vi "VI Auto Kalibrieren.vi"() -> ()   [LabVIEW 2020, in "Auto Kalibrieren.lvlib"]
uses:
  Auto Kalibrieren.lvlib
  Visualisierungs Elemente/Button.ctl
  Visualisierungs Elemente/String - Ausgabefeld.ctl
  Visualisierungs Elemente/Zahlen-Ausgabefeld.ctl
  Funktionstasten/Funktionstasten-Aktion.ctl
  Funktionstasten/Zustaende.ctl
  Aktionen FGV Zustand Kalibrierung.ctl
  Funktionstasten/Freigabe Aktionen.ctl
  Seiten/FT-IR/FGV FT-IR Gasliste Aktionen.ctl
  Aktionen Timeout.ctl
  Analysator Definition/FGV Analysator Definition Aktionen.ctl
  Status Analysatoren/Aktion Status Analysatoren.ctl
  Aktion FGV CalZustand.ctl
  Seiten/CalGas Aufschaltung/FGV CalGas Aktionen.ctl
  Funktionstasten/Aktionen Zustaende Loggen.ctl
  Sprachverwaltung/FGV Aktion Tabelle zerlegen.ctl
  Aktion FGV Autokal GT.ctl
  Aktionen FID kalibrieren.ctl
  Aktionen FT-IR Kalibrieren.ctl
  Seiten/FT-IR/TOOLweb Interface Library/Trigger Aktionen.ctl
  Aktionen PMA kalibrieren.ctl
  Messdaten/Aktionen FGV Messdaten.ctl
  Seiten/EL3000/Allgemeine VI/FGV Uras26 Aktion.ctl
  Aktionen Zeitstempel speichern.ctl
  Stoerungen/FGV Stoerung aufnehmen Aktion.ctl
  Seiten/FT-IR/ReadLabFile/Aktionen Lab File.ctl
  Stoerungen/Stoerungen Messgeraet/Aktionen Kommunikation Stoerung.ctl
  SysLog/SysLog Interface.ctl
  Seiten/FT-IR/TOOLweb Interface Library/TOOLweb Interface.lvlib
  Seiten/FT-IR/TOOLweb Interface Library/Typdefinitionen.lvlib
  Funktionstasten/Funktionstasten.lvlib
  Allgemein/allgemeine Sub-VIs.lvlib
  Seiten/FT-IR/FT-IR.lvlib
  Messdaten/Messdaten.lvlib
  Analysator Definition/Analysator Definition.lvlib
  Seiten/EL3000/PMA/Kalibrieren/Kalibrieren.lvlib
  Seiten/EL3000/Allgemeine VI/Allgemeine VI.lvlib
  Status Analysatoren/Status Analysatoren.lvlib
  Seiten/EL3000/FID/FID Kalibrierung/FID Kalibrierung.lvlib
  Seiten/CalGas Aufschaltung/CalGas Aufschaltung.lvlib
  SysLog/SysLog.lvlib
  Stoerungen/Stoerungen.lvlib
  Seiten/FT-IR/ReadLabFile/Read Lab File.lvlib
  Linearisierung V2/Linearisierung v2.lvlib
  Sprachverwaltung/Sprachverwaltung.lvlib
panel:
  out "Endpunktgas Konzentration O2:":T1 caption="%" format="%.2f"
  out "Endpunktgas Konzentration THC:":T1 caption="ppm" format="%.2f"
  out "Zustand FID THC":T2
  out "Dev THC":sgl caption="ppm" format="%.2f"
  out "Rohwert THC":T1 caption="ppm" format="%.2f"
  out "Dev CH4":sgl caption="ppm" format="%.2f"
  out "Raw value CH4":T1 caption="ppm" format="%.2f"
  out "Zustand FID":T2
  out "Zustand PMA":T2
  out "Dev O2":sgl caption="Konzentration" format="%.2f"
  out "Rohwert O2":T1 caption="%" format="%.2f"
  out "Zustand FT-IR":T2
  out "Dev H2O":sgl caption="Konzentration" format="%.2f"
  out "Dev CO2":sgl caption="Konzentration" format="%.2f"
  out "CO2":T1 caption="%" format="%.2f"
  out "H2O":T1 caption="%" format="%.2f"
  out "Zeit:":T1 caption="Zeit"
  in  "ABBRECHEN":T3
  # "Auto Kalibrierung"
  # "sec"
  # "FID CH4:"
  # "FID THC:"
  # "Dev.:"
  # "Dev.:"
  # "Dev.:"
  # "%"
  # "PMD:"
  # "Dev.:"
  # "%"
  # "Dev.:"
  # "%"
  # "FT-IR:"
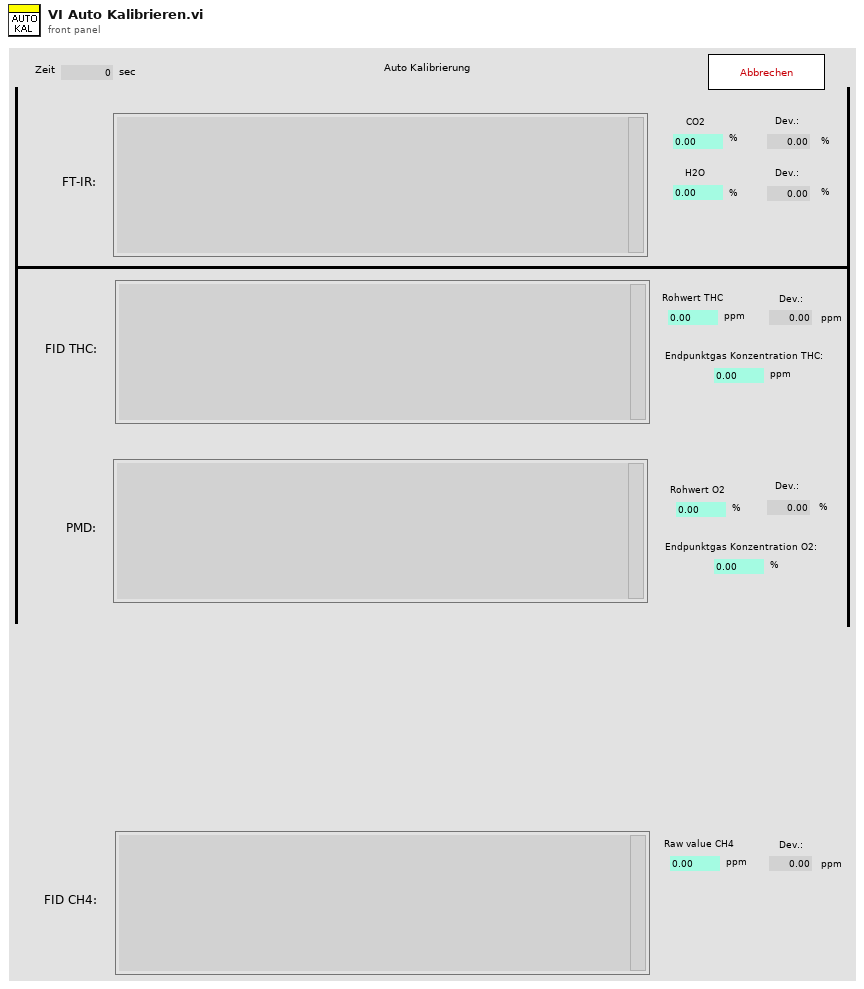
[diagram p1: front panel]
types:
  T1 = typedef "Zahlen-Ausgabefeld.ctl" = sgl
  T2 = typedef "String - Ausgabefeld.ctl" = string
  T3 = typedef "Button.ctl" = bool
  T4 = typedef "Funktionstasten.lvlib/Zustaende.ctl" = enum16{"Standby", "Pause", "Eco", "Messen", "Kalibrieren", "Spülen Filter", "Spülen Leitung", "Umgebungsluft", "0-Gas", "Cal-Gas", "CG zu PNS", "-------------", "Init 1", "Init 2", "Init 3", "Init 4", "Messen vorbereiten", "Messen durchführen", "Exit"}
  T5 = typedef "Funktionstasten.lvlib/Funktionstasten-Aktion.ctl" = enum16{"Initialisieren", "Zustand setzen", "Taste gedrückt", "Fehler speichern", "Lesen", "Manuell", "Remote", "Bitparallel", "Samplepoint", "Zeit Prüfen", "reset Umschalten"}
  T6 = typedef "Sprachverwaltung.lvlib/FGV Aktion Tabelle zerlegen.ctl" = enum16{"laden", "vereinzeln", "speichern"}
  T7 = typedef "Funktionstasten.lvlib/Aktionen Zustaende Loggen.ctl" = enum16{"lesen", "schreiben", "löschen", "init"}
  T8 = typedef "CalGas Aufschaltung.lvlib/FGV CalGas Aktionen.ctl" = enum16{"lesen", "Analysator Auswahl", "Def.CalGas", "Aufschaltung CalGas", "laden", "speichern", "KAL extrahieren"}
  T9 = typedef "Auto Kalibrieren.lvlib/Aktion FGV CalZustand.ctl" = enum16{"lesen", "Cal FTIR", "Cal FID CH4", "Cal PMA", "init", "Cal FID THC", "THC CG Eingang"}
  T10 = typedef "Status Analysatoren.lvlib/Aktion Status Analysatoren.ctl" = enum16{"lesen", "initialisieren", "Analysatoren aktiv", "FTIR Fehler", "FID Fehler", "PMA Fehler", "Felder einfärben"}
  T11 = typedef "Analysator Definition.lvlib/FGV Analysator Definition Aktionen.ctl" = enum16{"lesen", "MB setzen", "MB KAL setzen", "laden"}
  T12 = typedef "Auto Kalibrieren.lvlib/Aktionen Timeout.ctl" = enum16{"lesen", "init", "prüfen"}
  T13 = typedef "FT-IR.lvlib/FGV FT-IR Gasliste Aktionen.ctl" = enum16{"lesen", "Gasliste FT-IR", "Gasliste ausgelesen", "laden", "speichern", "löschen"}
  T14 = typedef "Funktionstasten.lvlib/Freigabe Aktionen.ctl" = enum16{"prüfen", "Freigabe?", "lesen"}
  T15 = typedef "Auto Kalibrieren.lvlib/Aktionen FGV Zustand Kalibrierung.ctl" = enum16{"lesen", "LÖSCHEN", "Hintergrund fertig", "Nullpunkt NDIR CO lo", "Endpunkt NDIR CO lo", "Nullpunkt NDIR CO hi", "Endpunkt NDIR CO hi", "Nullpunkt NDIR CO2 lo", "Endpunkt NDIR CO2 lo", "Nullpunkt FID CH4", "Endpunkt FID CH4", "Nullpunkt FID THC", "Endpunkt FID THC", "Nullpunkt PMA", "Endpunkt PMA", "Fehler FT-IR", "Fehler NDIR lo", "Fehler FID CH4", "Fehler FID THC", "Fehler PMA", "TIMEOUT"}
  T16 = typedef "Auto Kalibrieren.lvlib/Aktion FGV Autokal GT.ctl" = enum16{"lesen", "Autokal GT", "Referenz Start"}
  T17 = typedef "Status Analysatoren.lvlib/Status.ctl" = cluster{"FT-IR aktiv":bool, "FT-IR Fehler":bool, "FID aktiv":bool, "FID Fehler":bool, "PMA aktiv":bool, "PMA Fehler":bool}
  T18 = typedef "Analysator Definition.lvlib/Betriebsdaten Komponente.ctl" = cluster{"Namen":string[], "MB Namen":string[], "Einheit":string, "MB Aktuell":u16, "MB Endwert":u16, "CalGase":u16[], "MB für KAL":u16[], "CG für KAL":u16[]}
  T19 = typedef "ABB-EL3000.lvlib/Allgemeine VI.lvlib/FGV Uras26 Aktion.ctl" = enum16{"lesen", "CAL-Daten laden", "Messen", "Kalibrieren vorbereiten", "Kalibrieren", "CAL-Daten speichern", "Toleranz schreiben", "CAL-Daten kopieren"}
  T20 = typedef "Messdaten.lvlib/Aktionen FGV Messdaten.ctl" = enum16{"lesen", "schreiben", "löschen", "Mittelwerte", "Komponente"}
  T21 = typedef "Auto Kalibrieren.lvlib/Aktionen Zeitstempel speichern.ctl" = enum16{"lesen", "Zeitstempel NEU", "laden", "speichern"}
  T22 = typedef "CalGas Aufschaltung.lvlib/Definition CalGas Anzeige.ctl" = cluster{"Namen":T23, "Werte":T25, "Werte 2":T25, "Einheit":T27, "Messbereiche":T29}
  T23 = typedef "CalGas Aufschaltung.lvlib/CalGas-Namen.ctl" = cluster{"Name":T24, "Name 2":T24, "Name 3":T24, "Name 4":T24, "Name 5":T24, "Name 6":T24, "Name 7":T24, "Name 8":T24, "Name 9":T24, "Name 10":T24, "Name 11":T24, "Name 12":T24}
  T24 = typedef "String - Eingabefeld.ctl" = string
  T25 = typedef "CalGas Aufschaltung.lvlib/CalGas-Werte.ctl" = cluster{"Konzentration 1":T26, "Konzentration 2":T26, "Konzentration 3":T26, "Konzentration 4":T26, "Konzentration 5":T26, "Konzentration 6":T26, "Konzentration 7":T26, "Konzentration 8":T26, "Konzentration 9":T26, "Konzentration 10":T26, "Konzentration 11":T26, "Konzentration 12":T26}
  T26 = typedef "Zahlen-Eingabefeld.ctl" = sgl
  T27 = typedef "CalGas Aufschaltung.lvlib/CalGas-Einheit.ctl" = cluster{"Einheit 1":T28, "Einheit 2":T28, "Einheit 3":T28, "Einheit 4":T28, "Einheit 5":T28, "Einheit 6":T28, "Einheit 7":T28, "Einheit 8":T28, "Einheit 9":T28, "Einheit 10":T28, "Einheit 11":T28, "Einheit 12":T28}
  T28 = typedef "Auswahlfeld.ctl" = u16
  T29 = typedef "CalGas Aufschaltung.lvlib/CalGas-Messbereiche.ctl" = cluster{"Messbereich 1":T28, "Messbereich 2":T28, "Messbereich 3":T28, "Messbereich 4":T28, "Messbereich 5":T28, "Messbereich 6":T28, "Messbereich 7":T28, "Messbereich 8":T28, "Messbereich 9":T28, "Messbereich 10":T28, "Messbereich 11":T28, "Messbereich 12":T28}
  T30 = typedef "FT-IR.lvlib/TOOLweb Interface.lvlib/Typdefinitionen.lvlib/Trigger Aktionen.ctl" = enum16{"startrun", "runonce", "stoprun", "pauserun", "resumerun", "takeback"}
  T31 = typedef "Auto Kalibrieren.lvlib/Aktionen FT-IR Kalibrieren.ctl" = enum16{"Initialisieren", "Anstehende Störung", "CO2, H2O - Vergleichen", "Hintergrund starten", "Hintergrund", "Hintergrund Abgeschlossen", "Fertig", "Beenden"}
  T32 = typedef "Auto Kalibrieren.lvlib/Zustand Messgeraete Kalibrierung.ctl" = cluster{"Hintergrund FT-IR":bool, "Nullpunkt NDIR CO lo":bool, "Endpunkt NDIR CO lo":bool, "Nullpunkt NDIR CO hi":bool, "Endpunkt NDIR CO hi":bool, "Nullpunkt NDIR CO2 lo":bool, "Endpunkt NDIR CO2 lo":bool, "Nullpunkt FID CH4":bool, "Endpunkt FID CH4":bool, "Nullpunkt FID THC":bool, "Endpunkt FID THC":bool, "Nullpunkt PMA":bool, "Endpunkt PMA":bool, "Fehler FT-IR":bool, "Fehler NDIR lo":bool, "Fehler FID CH4":bool, "Fehler FID THC":bool, "Fehler PMA":bool}
  T33 = cluster{"action-name":string, "lastname":string, "lastdatetime":timestamp, "Systemzeit":timestamp}
  T34 = typedef "Auto Kalibrieren.lvlib/Aktionen PMA kalibrieren.ctl" = enum16{"Initialisieren", "Warten auf FT-IR", "Anstehende Störung", "0-Gas Aufschalten", "Nullpunkt Anfordern", "Nullpunkt", "Warten auf andere Messgeräte", "Messgas Aufschalten", "Endpunkt Anfordern", "Endpunkt", "Fertig", "Speichern"}
  T35 = typedef "Auto Kalibrieren.lvlib/Aktionen FID kalibrieren.ctl" = enum16{"Initialisieren", "Warten auf FTIR", "Anstehende Störung", "0-Gas Aufschalten", "Nullpunkt Anfordern", "Nullpunkt", "Warten auf andere Messgeräte", "Messgas Aufschalten", "Endpunkt Anfordern", "Endpunkt", "Endpunkt kopieren", "Fertig", "Speichern"}
  T36 = typedef "SysLog.lvlib/SysLog Interface.ctl" = cluster{"FehlermeldungsCode":i32, "ErfolgsmeldungsCode":i32, "ParameterListenString":string, "Anzeige":bool, "SysLogIcon":enum16{"OK", "Warnung", "Fehler"}, "intern":bool}
  T37 = typedef "Stoerungen.lvlib/FGV Stoerung aufnehmen Aktion.ctl" = enum16{"Initialisieren", "Schreiben", "Lesen", "Quittieren", "quit. löschen"}
  T38 = typedef "FT-IR.lvlib/Read Lab File.lvlib/Aktionen Lab File.ctl" = enum16{"lesen", "laden"}
  T39 = typedef "Stoerungen.lvlib/Aktionen Kommunikation Stoerung.ctl" = enum16{"lesen", "init", "FT-IR Komm", "FT-IR Betriebsart", "FT-IR Hintergrund", "cRIO Komm", "PNS Komm", "Dichtheitstest", "Life Bit", "FTIR Komm AK", "PMA Komm", "FID Komm", "PMA Cal", "FID Ch4 Cal", "FID THC Cal", "Cal Timeout", "VFS 1 Komm", "VFS 2 Komm", "VFS 3 Komm", "VFS 4 Komm", "TRE 08 Komm", "CG-Test vorzeitig", "CG-Test Span 1", "CG-Test Span 2", "CG-Test Span 3", "CG-Test Messgas", "CG-Test löschen", "Test", "Amium AK", "AK Recept konfig", "AK Name konfig", "AK EKFG konfig"}
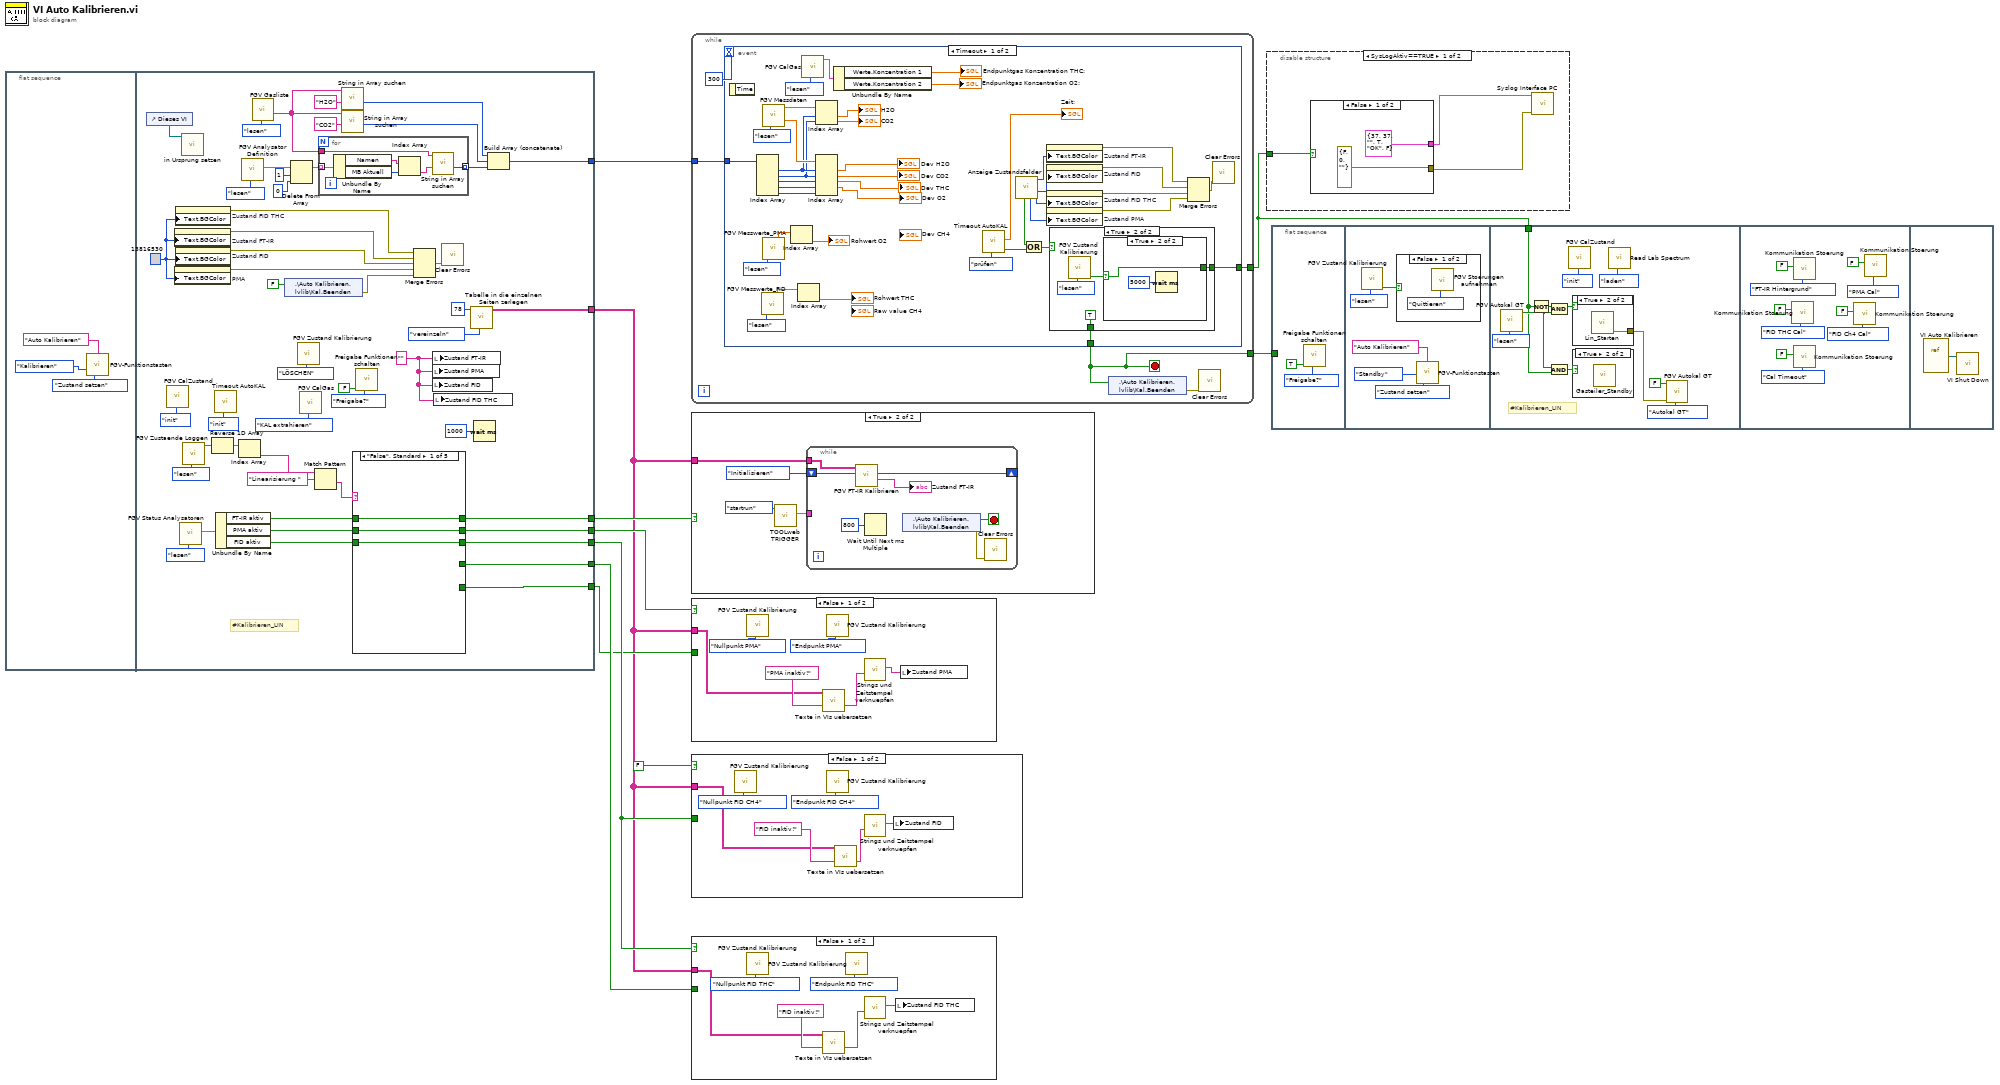
[diagram p0: block diagram]
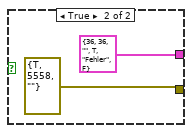
[diagram p2: hidden frame]
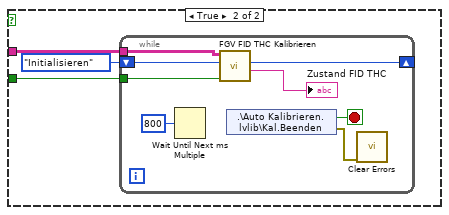
[diagram p4: hidden frame]
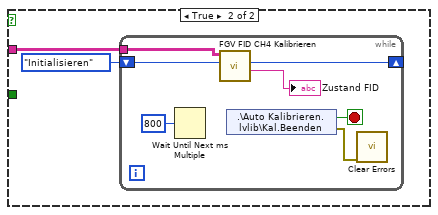
[diagram p5: hidden frame]
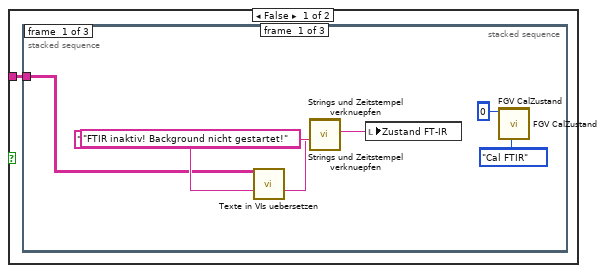
[diagram p6: hidden frame]
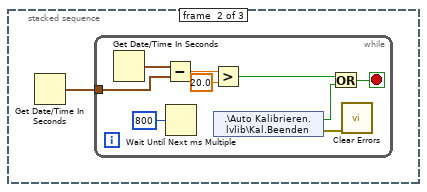
[diagram p7: hidden frame]
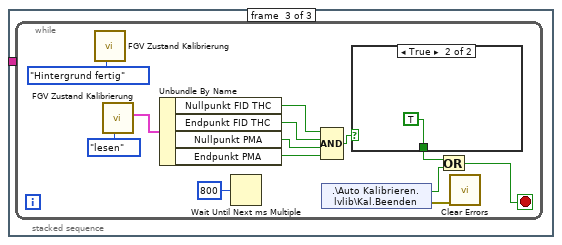
[diagram p8: hidden frame]
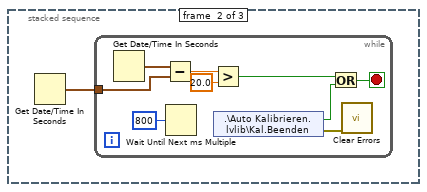
[diagram p10: hidden frame]
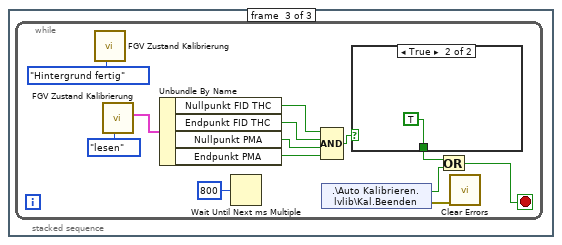
[diagram p11: hidden frame]
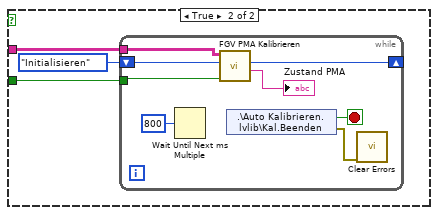
[diagram p13: hidden frame]
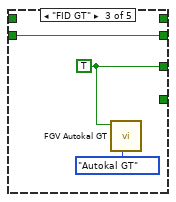
[diagram p18: hidden frame]
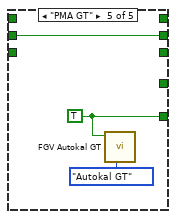
[diagram p20: hidden frame]
diagram:
  n1 = flat-sequence {
    tunnel: [w42] -> w9
    tunnel: [w28] -> w5
    tunnel: [w31] -> w8
    tunnel: [w26] -> w6
    tunnel: [w19] -> w4
    tunnel: [w18] -> w3
    tunnel: [w15] -> w1
    frame #0 {
      n2 = call "FGV-Funktionstasten.vi"("Herkunft"="Auto Kalibrieren", "Zustand"=Zustaende."Kalibrieren", "Aktion"=Funktionstasten-Aktion."Zustand setzen") -> ()  [unwired: 5 in, 8 out]
    }
    frame #1 {
      w33 = u32 13816530 ("Farbfeld")
      w35 = T2 "" ("Zustand FT-IR")
      # "#Kalibrieren_LIN"
      n3 = control-ref of="Dieses VI"() -> (w14:refnum<vi>)
      n4 = call "FGV CalZustand.vi"("Aktion"=Aktion_FGV_CalZustand."init") -> ()  [unwired: 14 in, 5 out]
      n5 = property on="Zustand FT-IR" class="Str (strikt)"("Text.BGColor"=w33) -> (error out=w52:errorcluster)  [unwired: 2 in, 1 out]
      n6 = property on="PMA" class="Str (strikt)"("Text.BGColor"=w33) -> (error out=w54:errorcluster)  [unwired: 2 in, 1 out]
      n7 = property on="Zustand FID THC" class="Str (strikt)"("Text.BGColor"=w33) -> (error out=w34:errorcluster)  [unwired: 2 in, 1 out]
      n8 = property on="Zustand FID" class="Str (strikt)"("Text.BGColor"=w33) -> (error out=w36:errorcluster)  [unwired: 2 in, 1 out]
      n9 = call "FGV Status Analysatoren.vi"("Aktionen"=Aktion_Status_Analysatoren."lesen") -> ("Status Analysatoren"=w38:T17)  [unwired: 10 in]
      n10 = call "in Ursprung setzen.vi"("VI Referenz"=w14) -> ()  [unwired: 10 in, 1 out]
      n11 = call "FGV Zustaende Loggen.vi"("Aktionen Zustände Loggen"=Aktionen_Zustaende_Loggen."lesen") -> ("Log Daten"=w21:string[])  [unwired: 9 in, 1 out]
      n12 = Reverse 1D Array(array=w21) -> (reversed array=w20:string[])
      n13 = call "Timeout AutoKAL.vi"("Aktionen"=Aktionen_Timeout."init") -> ()  [unwired: 9 in, 2 out]
      n14 = Unbundle By Name(w38) -> ("FT-IR aktiv"=w30:bool, "PMA aktiv"=w29:bool, "FID aktiv"=w27:bool)
      n15 = Index Array(array=w20) -> (element=w24:string)  [unwired: 1 in]
      n16 = call "FGV Analysator Definition.vi"("Aktionen"=FGV_Analysator_Definition_Aktionen."lesen") -> ("Betriebsdaten"=w50:T18[])  [unwired: 6 in, 4 out]
      n17 = call "FGV Gasliste.vi"("Aktionen"=FGV_FT-IR_Gasliste_Aktionen."lesen") -> ("Aktuelle Gasliste gesamt"=w46:T2[])  [unwired: 8 in, 2 out]
      n18 = shared-variable ".\\Auto Kalibrieren.lvlib\\Kal.Beenden"(FALSE ("Kal.Beenden")) -> (error out=w40:errorcluster)  [unwired: 1 in]
      n19 = Delete From Array(array=w50, length=1 ("Länge"), index=0 ("Index")) -> (array with subset deleted=w47:T18[])  [unwired: 1 out]
      n20 = call "FGV Zustand Kalibrierung.vi"("Aktionen"=Aktionen_FGV_Zustand_Kalibrierung."LÖSCHEN" ("Enum")) -> ()  [unwired: 9 in, 2 out]
      n21 = call "FGV CalGas.vi"("Aktionen"=FGV_CalGas_Aktionen."KAL extrahieren") -> ()  [unwired: 6 in, 5 out]
      n22 = Match Pattern(string=w24, regular expression="Linearisierung " ("Regulärer Ausdruck")) -> (after substring=w22:string)  [unwired: 1 in, 3 out]
      n23 = for {
        tunnel: w47 -> [w79] mode=indexing
        tunnel: w46 -> [w75]
        tunnel: [w74] -> w43 mode=indexing
        n24 = Unbundle By Name(w79) -> ("Namen"=w77:string[], "MB Aktuell"=w78:u16)
        n25 = Index Array(array=w77, index=w78) -> (element=w76:string)
        n26 = call "String in Array suchen.vi"("Nach String/Zeichen suchen (-)"=w76, "String-Array"=w75) -> ("Index"=w74:i32)  [unwired: 7 in, 2 out]
      }
      n27 = call "String in Array suchen.vi"("Nach String/Zeichen suchen (-)"="H2O", "String-Array"=w46) -> ("Index"=w45:i32)  [unwired: 7 in, 2 out]
      n28 = call "String in Array suchen.vi"("Nach String/Zeichen suchen (-)"="CO2", "String-Array"=w46) -> ("Index"=w44:i32)  [unwired: 7 in, 2 out]
      n29 = case shown="\"False\", Standard" w22 {
        tunnel: [w65 _ _ _ _] -> w31
        tunnel: w30 -> [w65 _ _ _ _]
        tunnel: w29 -> [w64 _ _ w70 w73]
        tunnel: [w64 _ _ w70 w73] -> w28
        tunnel: w27 -> [w63 w66 w69 _ _]
        tunnel: [w63 w66 w69 _ _] -> w26
        tunnel: [_ _ w68 _ _] -> w19
        tunnel: [_ _ _ _ w71] -> w18
        frame "False", Default {
        }
        frame "FID" {
        }
        frame "FID GT" {
          w68 = TRUE
          n30 = call "FGV Autokal GT.vi"("Aktion FGV AutoKal"=Aktion_FGV_Autokal_GT."Autokal GT", "Autokal GT Aktiv?"=w68) -> ()  [unwired: 7 in, 3 out]
        }
        frame "PMA" {
        }
        frame "PMA GT" {
          w71 = TRUE
          n31 = call "FGV Autokal GT.vi"("Aktion FGV AutoKal"=Aktion_FGV_Autokal_GT."Autokal GT", "Autokal GT Aktiv?"=w71) -> ()  [unwired: 7 in, 3 out]
        }
      }
      n32 = call "Freigabe Funktionen schalten.vi"("Aktionen"=Freigabe_Aktionen."Freigabe?", "Freigabe?"=FALSE) -> ()  [unwired: 7 in, 3 out]
      n33 = Merge Errors(w34, w52, w36, w54, w40) -> (w53:errorcluster)
      n34 = local write "Zustand PMA"(w35) -> ()
      n35 = local write "Zustand FID"(w35) -> ()
      n36 = local write "Zustand FT-IR"(w35) -> ()
      n37 = local write "Zustand FID THC"(w35) -> ()
      n38 = call <vilib>:"Clear Errors.vi"("error in (no error)"=w53) -> ()  [unwired: 5 in, 2 out]
      n39 = call "Tabelle in die einzelnen Seiten zerlegen.vi"("Aktion"=FGV_Aktion_Tabelle_zerlegen."vereinzeln", "Index (Seite)"=78) -> ("Sprachliste"=w15:string[][])  [unwired: 7 in, 2 out]
      n40 = Wait (ms)(milliseconds to wait=u32 1000 ("Zu wartende ms")) -> ()  [unwired: 1 out]
      n41 = Build Array (concatenate)(w45, w44, w43) -> (w42:i32[])
    }
  }
  n42 = while {
    tunnel: [w83] -> w10
    tunnel: w9 -> [w81]
    tunnel: [w80] -> w2
    stop <- w83 stop-if-true
    n43 = event shown="[0] Timeout" {
      selector: _ -> [_ _]
      dyn-events: _ -> [_ _]
      timeout: 300 -> [_ _]
      tunnel: [w124 TRUE ("ABBRECHEN")] -> w83
      tunnel: w81 -> [w107 _]
      tunnel: [w89 _] -> w80
      event Timeout {
        n44 = event-data() -> ()  [unwired: 1 in, 1 out]
        n45 = Index Array(array=w107) -> (element #1=w106:i32, element #2=w105:i32, element #3=w104:i32, element #4=w103:i32, element #5=w102:i32)  [unwired: 5 in]
        n46 = call "FGV Messwerte_FID.vi"("Aktion"=FGV_Uras26_Aktion."lesen") -> ("Rohwerte"=w99:sgl[])  [unwired: 19 in, 7 out]
        n47 = call "FGV Messdaten.vi"("Aktionen"=Aktionen_FGV_Messdaten."lesen") -> ("Aktuelle Messwerte"=w123:sgl[], "Deviation"=w119:sgl[])  [unwired: 6 in, 7 out]
        n48 = call "FGV Messwerte_PMA.vi"("Aktion"=FGV_Uras26_Aktion."lesen") -> ("Rohwerte"=w93:sgl[])  [unwired: 19 in, 7 out]
        n49 = Index Array(array=w93) -> (element=→"Rohwert O2":sgl)  [unwired: 1 in]
        n50 = Index Array(array=w99) -> (element=→"Rohwert THC":sgl)  [unwired: 1 in]
        n51 = call "FGV CalGas.vi"("Aktionen"=FGV_CalGas_Aktionen."lesen") -> ("Def.CalGas"=w87:T22)  [unwired: 6 in, 4 out]
        n52 = Index Array(array=w123, index #1=w106, index #2=w105) -> (element #1=→"H2O":sgl, element #2=→"CO2":sgl)
        n53 = Index Array(array=w119, index #1=w106, index #2=w105, index #3=w104, index #4=w103, index #5=w102) -> (element #1=→"Dev H2O":sgl, element #2=→"Dev CO2":sgl, element #3=→"Dev THC":sgl, element #4=→"Dev O2":sgl)  [unwired: 1 out]
        n54 = Unbundle By Name(w87) -> ("Werte.Konzentration 1"=→"Endpunktgas Konzentration THC:":T26, "Werte.Konzentration 2"=→"Endpunktgas Konzentration O2:":T26)
        n55 = call "Timeout AutoKAL.vi"("Aktionen"=Aktionen_Timeout."prüfen") -> ("Timeout"=w113:bool, "Verstrichene Zeit"=→"Zeit:":dbl)  [unwired: 9 in]
        n56 = call "Anzeige Zustandsfelder.vi"() -> ("Zustand FID THC"=w97:u32, "Zustand FID CH4"=w98:u32, "Zustand FT-IR"=w125:u32, "Zustand PMA"=w108:u32, "BEENDEN"=w114:bool)  [unwired: 6 in, 1 out]
        n57 = Or(x=w114, y=w113) -> (x .or. y?=w115:bool)
        n58 = property on="Zustand FT-IR" class="Str (strikt)"("Text.BGColor"=w125) -> (error out=w111:errorcluster)  [unwired: 2 in, 1 out]
        n59 = property on="Zustand FID" class="Str (strikt)"("Text.BGColor"=w98) -> (error out=w101:errorcluster)  [unwired: 2 in, 1 out]
        n60 = property on="Zustand FID THC" class="Str (strikt)"("Text.BGColor"=w97) -> (error out=w96:errorcluster)  [unwired: 2 in, 1 out]
        n61 = property on="Zustand PMA" class="Str (strikt)"("Text.BGColor"=w108) -> (error out=w109:errorcluster)  [unwired: 2 in, 1 out]
        n62 = case shown="True" w115 {
          tunnel: [_ TRUE] -> w124
          tunnel: [_ w126] -> w89
          frame False {
          }
          frame True {
            n63 = call "FGV Zustand Kalibrierung.vi"("Aktionen"=Aktionen_FGV_Zustand_Kalibrierung."lesen" ("Enum")) -> ("Fehler"=w127:bool)  [unwired: 9 in, 1 out]
            n64 = case shown="True" w127 {
              selector: w127 -> [_ w133]
              tunnel: [_ w133] -> w126
              frame False {
                n65 = stacked-sequence {
                  frame #0 {
                    (unwired) FALSE ("case")
                    n66 = call "Zeitstempel letzte Kalibrierungen.vi"("Aktionen"=Aktionen_Zeitstempel_speichern."Zeitstempel NEU") -> ()  [unwired: 10 in, 1 out]
                  }
                  frame #1 {
                    n67 = call "Zeitstempel letzte Kalibrierungen.vi"("Aktionen"=Aktionen_Zeitstempel_speichern."speichern") -> ()  [unwired: 10 in, 1 out]
                  }
                  frame #2 {
                    n68 = Wait (ms)(milliseconds to wait=u32 7000 ("Zu wartende ms")) -> ()  [unwired: 1 out]
                  }
                }
              }
              frame True {
                n69 = Wait (ms)(milliseconds to wait=u32 5000 ("Zu wartende ms")) -> ()  [unwired: 1 out]
              }
            }
          }
        }
        n70 = Merge Errors(w111, w101, w96, w109) -> (w110:errorcluster)
        n71 = call <vilib>:"Clear Errors.vi"("error in (no error)"=w110) -> ()  [unwired: 5 in, 2 out]
      }
      event Value Change {
        n72 = event-data() -> ()  [unwired: 1 in, 1 out]
      }
    }
    n73 = shared-variable ".\\Auto Kalibrieren.lvlib\\Kal.Beenden"(w83) -> (error out=w82:errorcluster)  [unwired: 1 in]
    n74 = call <vilib>:"Clear Errors.vi"("error in (no error)"=w82) -> ()  [unwired: 5 in, 2 out]
  }
  n75 = case shown="True" w8 {
    tunnel: w1 -> [w136 w195]
    frame False {
      n76 = stacked-sequence {
        tunnel: w136 -> [w137 _ _]
        frame #0 {
          n77 = call "Texte in VIs uebersetzen.vi"("Sprachliste"=w137, "String zum Übersetzen"="FTIR inaktiv! Background nicht gestartet!" ("String 1 hinzufügen")) -> ("String zum Übersetzen"=w138:string)  [unwired: 9 in, 4 out]
          n78 = call "Strings und Zeitstempel verknuepfen.vi"("String 1 hinzufügen"=w138) -> ("Verknüpfter String"=w142:string)  [unwired: 10 in]
          n79 = local write "Zustand FT-IR"(w142) -> ()
          n80 = call "FGV CalZustand.vi"("CAL Zustand"=u16 0 ("CAL Zustand FTIR"), "Aktion"=Aktion_FGV_CalZustand."Cal FTIR") -> ()  [unwired: 13 in, 5 out]
        }
        frame #1 {
          n81 = Get Date/Time In Seconds() -> (seconds since 1Jan1904=w143:timestamp)
          n82 = while {
            tunnel: w143 -> [w151]
            stop <- w145 stop-if-true
            n83 = Get Date/Time In Seconds() -> (seconds since 1Jan1904=w152:timestamp)
            n84 = Subtract(x=w152, y=w151) -> (x-y=w150:dbl)
            n85 = Wait Until Next ms Multiple(millisecond multiple=u32 800 ("Vielfache von ms")) -> ()  [unwired: 1 out]
            n86 = Greater?(x=w150, y=20.0) -> (0:w148:bool)
            n87 = shared-variable ".\\Auto Kalibrieren.lvlib\\Kal.Beenden"() -> (w146:bool, error out=w144:errorcluster)  [unwired: 1 in]
            n88 = Or(x=w148, y=w146) -> (x .or. y?=w145:bool)
            n89 = call <vilib>:"Clear Errors.vi"("error in (no error)"=w144) -> ()  [unwired: 5 in, 2 out]
          }
        }
        frame #2 {
          n90 = while {
            stop <- w154 stop-if-true
            n91 = call "FGV Zustand Kalibrierung.vi"("Aktionen"=Aktionen_FGV_Zustand_Kalibrierung."Hintergrund fertig" ("Enum")) -> ()  [unwired: 9 in, 2 out]
            n92 = call "FGV Zustand Kalibrierung.vi"("Aktionen"=Aktionen_FGV_Zustand_Kalibrierung."lesen" ("Enum")) -> ("Zustand Kalibrierung"=w163:T32)  [unwired: 9 in, 1 out]
            n93 = Unbundle By Name(w163) -> ("Nullpunkt FID THC"=w162:bool, "Endpunkt FID THC"=w161:bool, "Nullpunkt PMA"=w160:bool, "Endpunkt PMA"=w159:bool)
            n94 = Wait Until Next ms Multiple(millisecond multiple=u32 800 ("Vielfache von ms")) -> ()  [unwired: 1 out]
            n95 = Compound Arithmetic op=AND(w162, w161, w160, w159) -> (w158:bool)
            n96 = shared-variable ".\\Auto Kalibrieren.lvlib\\Kal.Beenden"() -> (w157:bool, error out=w156:errorcluster)  [unwired: 1 in]
            n97 = case shown="True" w158 {
              tunnel: [_ TRUE ("Nullpunkt FID")] -> w155
              frame False {
              }
              frame True {
              }
            }
            n98 = Or(x=w155, y=w157) -> (x .or. y?=w154:bool)
            n99 = call <vilib>:"Clear Errors.vi"("error in (no error)"=w156) -> ()  [unwired: 5 in, 2 out]
          }
        }
      }
      n100 = stacked-sequence {
        frame #0 {
          n101 = call "Strings und Zeitstempel verknuepfen.vi"("String 1 hinzufügen"="FTIR inaktive! Background nicht gestartet!") -> ("Verknüpfter String"=w169:string)  [unwired: 10 in]
          n102 = local write "Zustand FT-IR"(w169) -> ()
          n103 = call "FGV CalZustand.vi"("CAL Zustand"=u16 0 ("CAL Zustand FTIR"), "Aktion"=Aktion_FGV_CalZustand."Cal FTIR") -> ()  [unwired: 13 in, 5 out]
        }
        frame #1 {
          n104 = Get Date/Time In Seconds() -> (seconds since 1Jan1904=w171:timestamp)
          n105 = while {
            tunnel: w171 -> [w179]
            stop <- w173 stop-if-true
            n106 = Get Date/Time In Seconds() -> (seconds since 1Jan1904=w180:timestamp)
            n107 = Subtract(x=w180, y=w179) -> (x-y=w178:dbl)
            n108 = Wait Until Next ms Multiple(millisecond multiple=u32 800 ("Vielfache von ms")) -> ()  [unwired: 1 out]
            n109 = Greater?(x=w178, y=20.0) -> (0:w176:bool)
            n110 = shared-variable ".\\Auto Kalibrieren.lvlib\\Kal.Beenden"() -> (w174:bool, error out=w172:errorcluster)  [unwired: 1 in]
            n111 = Or(x=w176, y=w174) -> (x .or. y?=w173:bool)
            n112 = call <vilib>:"Clear Errors.vi"("error in (no error)"=w172) -> ()  [unwired: 5 in, 2 out]
          }
        }
        frame #2 {
          n113 = while {
            stop <- w182 stop-if-true
            n114 = call "FGV Zustand Kalibrierung.vi"("Aktionen"=Aktionen_FGV_Zustand_Kalibrierung."Hintergrund fertig" ("Enum")) -> ()  [unwired: 9 in, 2 out]
            n115 = call "FGV Zustand Kalibrierung.vi"("Aktionen"=Aktionen_FGV_Zustand_Kalibrierung."lesen" ("Enum")) -> ("Zustand Kalibrierung"=w191:T32)  [unwired: 9 in, 1 out]
            n116 = Unbundle By Name(w191) -> ("Nullpunkt FID THC"=w190:bool, "Endpunkt FID THC"=w189:bool, "Nullpunkt PMA"=w188:bool, "Endpunkt PMA"=w187:bool)
            n117 = Wait Until Next ms Multiple(millisecond multiple=u32 800 ("Vielfache von ms")) -> ()  [unwired: 1 out]
            n118 = Compound Arithmetic op=AND(w190, w189, w188, w187) -> (w186:bool)
            n119 = shared-variable ".\\Auto Kalibrieren.lvlib\\Kal.Beenden"() -> (w185:bool, error out=w184:errorcluster)  [unwired: 1 in]
            n120 = case shown="True" w186 {
              tunnel: [_ TRUE ("Nullpunkt FID")] -> w183
              frame False {
              }
              frame True {
              }
            }
            n121 = Or(x=w183, y=w185) -> (x .or. y?=w182:bool)
            n122 = call <vilib>:"Clear Errors.vi"("error in (no error)"=w184) -> ()  [unwired: 5 in, 2 out]
          }
        }
      }
    }
    frame True {
      n123 = call "TOOLweb TRIGGER.vi"("action"=Trigger_Aktionen."startrun") -> ("trigger-Diagnose"=w196:T33)  [unwired: 5 in, 1 out]
      n124 = while {
        shift-right: [w203] -> _
        shift-left: Aktionen_FT-IR_Kalibrieren."Initialisieren" ("Aktionen FT-IR Kalibrieren") -> [w204]
        tunnel: w196 -> [_]
        tunnel: w195 -> [w199]
        stop <- w205 stop-if-true
        n125 = call "FGV FT-IR Kalibrieren.vi"("Aktionen FT-IR Kalibrieren"=w204, "Sprachliste"=w199) -> ("Zustand FT-IR"=→"Zustand FT-IR":string, "Aktionen FT-IR Kalibrieren"=w203:T31)  [unwired: 8 in]
        n126 = Wait Until Next ms Multiple(millisecond multiple=u32 800 ("Vielfache von ms")) -> ()  [unwired: 1 out]
        n127 = shared-variable ".\\Auto Kalibrieren.lvlib\\Kal.Beenden"() -> (w205:bool, error out=w200:errorcluster)  [unwired: 1 in]
        n128 = call <vilib>:"Clear Errors.vi"("error in (no error)"=w200) -> ()  [unwired: 5 in, 2 out]
      }
    }
  }
  n129 = case shown="False" w5 {
    tunnel: w3 -> [_ w213]
    tunnel: w1 -> [w206 w212]
    frame False {
      n130 = call "FGV Zustand Kalibrierung.vi"("Aktionen"=Aktionen_FGV_Zustand_Kalibrierung."Nullpunkt PMA" ("Enum")) -> ()  [unwired: 9 in, 2 out]
      n131 = call "Texte in VIs uebersetzen.vi"("Sprachliste"=w206, "String zum Übersetzen"="PMA inaktiv!" ("String 1 hinzufügen")) -> ("String zum Übersetzen"=w207:string)  [unwired: 9 in, 4 out]
      n132 = call "FGV Zustand Kalibrierung.vi"("Aktionen"=Aktionen_FGV_Zustand_Kalibrierung."Endpunkt PMA" ("Enum")) -> ()  [unwired: 9 in, 2 out]
      n133 = call "Strings und Zeitstempel verknuepfen.vi"("String 1 hinzufügen"=w207) -> ("Verknüpfter String"=w211:string)  [unwired: 10 in]
      n134 = local write "Zustand PMA"(w211) -> ()
    }
    frame True {
      n135 = while {
        shift-right: [w218] -> _
        shift-left: Aktionen_PMA_kalibrieren."Initialisieren" ("Aktionen PMA kalibrieren") -> [w219]
        tunnel: w213 -> [w216]
        tunnel: w212 -> [w215]
        stop <- w222 stop-if-true
        n136 = Wait Until Next ms Multiple(millisecond multiple=u32 800 ("Vielfache von ms")) -> ()  [unwired: 1 out]
        n137 = call "FGV PMA Kalibrieren.vi"("GT?"=w216, "Aktionen PMA kalibrieren"=w219, "Sprachliste"=w215) -> ("Zustand PMA"=→"Zustand PMA":string, "Aktionen PMA kalibrieren"=w218:T34)  [unwired: 7 in]
        n138 = shared-variable ".\\Auto Kalibrieren.lvlib\\Kal.Beenden"() -> (w222:bool, error out=w220:errorcluster)  [unwired: 1 in]
        n139 = call <vilib>:"Clear Errors.vi"("error in (no error)"=w220) -> ()  [unwired: 5 in, 2 out]
      }
    }
  }
  n140 = case shown="False" FALSE {
    tunnel: w6 -> [_ _]
    tunnel: w1 -> [w223 w229]
    frame False {
      n141 = call "FGV Zustand Kalibrierung.vi"("Aktionen"=Aktionen_FGV_Zustand_Kalibrierung."Nullpunkt FID CH4" ("Enum")) -> ()  [unwired: 9 in, 2 out]
      n142 = call "FGV Zustand Kalibrierung.vi"("Aktionen"=Aktionen_FGV_Zustand_Kalibrierung."Endpunkt FID CH4" ("Enum")) -> ()  [unwired: 9 in, 2 out]
      n143 = call "Texte in VIs uebersetzen.vi"("Sprachliste"=w223, "String zum Übersetzen"="FID inaktiv!" ("String 1 hinzufügen")) -> ("String zum Übersetzen"=w224:string)  [unwired: 9 in, 4 out]
      n144 = call "Strings und Zeitstempel verknuepfen.vi"("String 1 hinzufügen"=w224) -> ("Verknüpfter String"=w226:string)  [unwired: 10 in]
      n145 = local write "Zustand FID"(w226) -> ()
    }
    frame True {
      n146 = while {
        shift-right: [w233] -> _
        shift-left: Aktionen_FID_kalibrieren."Initialisieren" ("Aktionen FID kalibrieren") -> [w234]
        tunnel: w229 -> [w231]
        stop <- w237 stop-if-true
        n147 = Wait Until Next ms Multiple(millisecond multiple=u32 800 ("Vielfache von ms")) -> ()  [unwired: 1 out]
        n148 = call "FGV FID CH4 Kalibrieren.vi"("Aktionen FID kalibrieren"=w234, "Sprachliste"=w231) -> ("Zustand PMA"=→"Zustand FID":string, "Aktionen FID kalibrieren"=w233:T35)  [unwired: 8 in]
        n149 = shared-variable ".\\Auto Kalibrieren.lvlib\\Kal.Beenden"() -> (w237:bool, error out=w235:errorcluster)  [unwired: 1 in]
        n150 = call <vilib>:"Clear Errors.vi"("error in (no error)"=w235) -> ()  [unwired: 5 in, 2 out]
      }
    }
  }
  n151 = case shown="False" w6 {
    tunnel: w4 -> [_ w245]
    tunnel: w1 -> [w238 w244]
    frame False {
      n152 = call "FGV Zustand Kalibrierung.vi"("Aktionen"=Aktionen_FGV_Zustand_Kalibrierung."Nullpunkt FID THC" ("Enum")) -> ()  [unwired: 9 in, 2 out]
      n153 = call "Texte in VIs uebersetzen.vi"("Sprachliste"=w238, "String zum Übersetzen"="FID inaktiv!" ("String 1 hinzufügen")) -> ("String zum Übersetzen"=w239:string)  [unwired: 9 in, 4 out]
      n154 = call "FGV Zustand Kalibrierung.vi"("Aktionen"=Aktionen_FGV_Zustand_Kalibrierung."Endpunkt FID THC" ("Enum")) -> ()  [unwired: 9 in, 2 out]
      n155 = call "Strings und Zeitstempel verknuepfen.vi"("String 1 hinzufügen"=w239) -> ("Verknüpfter String"=w241:string)  [unwired: 10 in]
      n156 = local write "Zustand FID THC"(w241) -> ()
    }
    frame True {
      n157 = while {
        shift-right: [w250] -> _
        shift-left: Aktionen_FID_kalibrieren."Initialisieren" ("Aktionen FID kalibrieren") -> [w251]
        tunnel: w245 -> [w248]
        tunnel: w244 -> [w247]
        stop <- w254 stop-if-true
        n158 = Wait Until Next ms Multiple(millisecond multiple=u32 800 ("Vielfache von ms")) -> ()  [unwired: 1 out]
        n159 = call "FGV FID THC Kalibrieren.vi"("GT?"=w248, "Aktionen FID kalibrieren"=w251, "Sprachliste"=w247) -> ("Zustand"=→"Zustand FID THC":string, "Aktionen FID kalibrieren"=w250:T35)  [unwired: 7 in]
        n160 = shared-variable ".\\Auto Kalibrieren.lvlib\\Kal.Beenden"() -> (w254:bool, error out=w252:errorcluster)  [unwired: 1 in]
        n161 = call <vilib>:"Clear Errors.vi"("error in (no error)"=w252) -> ()  [unwired: 5 in, 2 out]
      }
    }
  }
  n162 = disable-structure shown="SysLogAktiv==TRUE" {
    disable-tunnel: w2 -> [w256 _]
    frame condition #0 (active) {
      n163 = case shown="False" w256 {
        tunnel: [errorcluster {"status"=FALSE, "code"=0, "source"=""} ("Fehler (in)") errorcluster {"status"=TRUE, "code"=5558, "source"=""} ("Fehler (in)")] -> w257
        tunnel: [T36 {"FehlermeldungsCode"=37, "ErfolgsmeldungsCode"=37, "ParameterListenString"="", "Anzeige"=TRUE, "SysLogIcon"=enum."OK", "intern"=FALSE} ("Cluster (in)") T36 {"FehlermeldungsCode"=36, "ErfolgsmeldungsCode"=36, "ParameterListenString"="", "Anzeige"=TRUE, "SysLogIcon"=enum."Fehler", "intern"=FALSE} ("Cluster (in)")] -> w255
        frame False {
        }
        frame True {
        }
      }
      n164 = call "Syslog Interface PC.vi"("Fehler (in)"=w257, "Cluster (in)"=w255) -> ()  [unwired: 9 in, 1 out]
    }
    frame condition #1 {
    }
  }
  n165 = flat-sequence {
    tunnel: w10 -> [_]
    tunnel: w2 -> [w271]
    frame #0 {
      n166 = call "Freigabe Funktionen schalten.vi"("Aktionen"=Freigabe_Aktionen."Freigabe?", "Freigabe?"=TRUE) -> ()  [unwired: 7 in, 3 out]
    }
    frame #1 {
      n167 = call "FGV Zustand Kalibrierung.vi"("Aktionen"=Aktionen_FGV_Zustand_Kalibrierung."lesen" ("Enum")) -> ("Fehler"=w264:bool)  [unwired: 9 in, 1 out]
      n168 = case shown="False" w264 {
        frame False {
          n169 = call "FGV Stoerungen aufnehmen.vi"("FGV Störung aufnehmen Aktion"=FGV_Stoerung_aufnehmen_Aktion."Quittieren") -> ()  [unwired: 7 in, 4 out]
        }
        frame True {
        }
      }
      n170 = call "FGV-Funktionstasten.vi"("Herkunft"="Auto Kalibrieren", "Zustand"=Zustaende."Standby", "Aktion"=Funktionstasten-Aktion."Zustand setzen") -> ()  [unwired: 5 in, 8 out]
    }
    frame #2 {
      # "#Kalibrieren_LIN"
      n171 = call "FGV Autokal GT.vi"("Aktion FGV AutoKal"=Aktion_FGV_Autokal_GT."lesen") -> ("Autokal GT Aktiv?"=w273:bool)  [unwired: 8 in, 2 out]
      n172 = Not(x=w271) -> (.not. x?=w276:bool)
      n173 = And(x=w276, y=w273) -> (x .and. y?=w277:bool)
      n174 = And(x=w273, y=w271) -> (x .and. y?=w272:bool)
      n175 = call "FGV CalZustand.vi"("Aktion"=Aktion_FGV_CalZustand."init") -> ()  [unwired: 14 in, 5 out]
      n176 = case shown="True" w277 {
        tunnel: [_ w281] -> w270
        frame False {
        }
        frame True {
          n177 = call "Lin_Starten.vi"() -> ("error out"=w281:errorcluster)  [unwired: 11 in]
        }
      }
      n178 = case shown="True" w272 {
        frame False {
        }
        frame True {
          n179 = call "Gasteiler_Standby.vi"() -> ()  [unwired: 12 in]
        }
      }
      n180 = call "Read Lab Spectrum.VI"("Aktionen"=Aktionen_Lab_File."laden") -> ()  [unwired: 7 in, 4 out]
      n181 = call "FGV Autokal GT.vi"("Aktion FGV AutoKal"=Aktion_FGV_Autokal_GT."Autokal GT", "error in (no error)"=w270, "Autokal GT Aktiv?"=FALSE) -> ()  [unwired: 6 in, 3 out]
    }
    frame #3 {
      n182 = call "Kommunikation Stoerung.vi"("Aktionen"=Aktionen_Kommunikation_Stoerung."FID THC Cal", "ERROR"=FALSE) -> ()  [unwired: 9 in, 1 out]
      n183 = call "Kommunikation Stoerung.vi"("Aktionen"=Aktionen_Kommunikation_Stoerung."Cal Timeout", "ERROR"=FALSE) -> ()  [unwired: 9 in, 1 out]
      n184 = call "Kommunikation Stoerung.vi"("Aktionen"=Aktionen_Kommunikation_Stoerung."FT-IR Hintergrund", "ERROR"=FALSE) -> ()  [unwired: 9 in, 1 out]
      n185 = call "Kommunikation Stoerung.vi"("Aktionen"=Aktionen_Kommunikation_Stoerung."FID Ch4 Cal", "ERROR"=FALSE) -> ()  [unwired: 9 in, 1 out]
      n186 = call "Kommunikation Stoerung.vi"("Aktionen"=Aktionen_Kommunikation_Stoerung."PMA Cal", "ERROR"=FALSE) -> ()  [unwired: 9 in, 1 out]
    }
    frame #4 {
      n187 = vi-ref "VI Auto Kalibrieren.vi"() -> (w292:refnum<vi>)
      n188 = call "VI Shut Down.vi"("VI Referenz"=w292) -> ()  [unwired: 11 in]
    }
  }
